vi "UDP Discover (subnet).vi"(0 "Name":string, 5 "receiver port":u16=10000, 7 "Excludes":string[](array[string]), 11 "error in (no error)":errorcluster) -> (4 "address:port":string, 6 "Address":string, 8 "Port":i32, 14 "local address":string, 15 "error out":errorcluster)   [LabVIEW 2020]
panel:
  in  "timeout ms (500)":i32=500
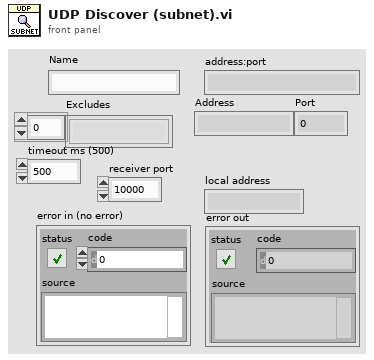
[diagram p1: front panel]
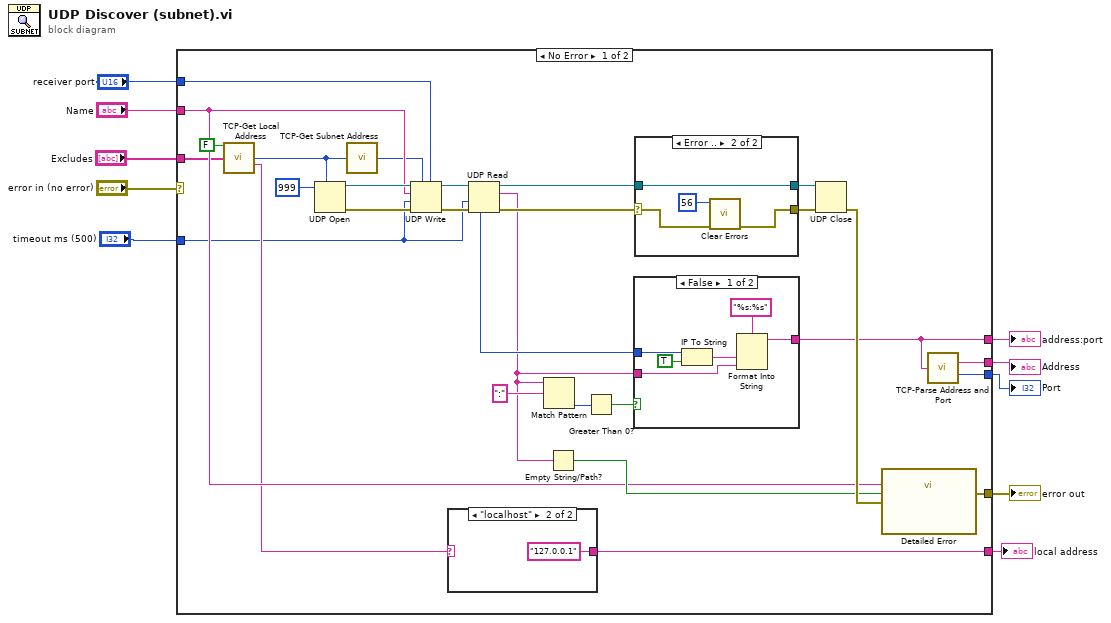
[diagram p0: block diagram]
diagram:
  n1 = case shown="No Error" "error in (no error)" {
    selector: "error in (no error)" -> [_ w55]
    tunnel: "receiver port" -> [w39 _]
    tunnel: [w24 _] -> w9
    tunnel: "Name" -> [w26 _]
    tunnel: [w25 w55] -> w7
    tunnel: [w23 _] -> w5
    tunnel: [w22 _] -> w4
    tunnel: [w20 _] -> w3
    tunnel: "Excludes" -> [w19 _]
    tunnel: "timeout ms (500)" -> [w11 _]
    frame No Error {
      n2 = call "TCP-Get Local Address.vi"("LAN first"=FALSE, "Excludes"=w19) -> ("net address"=w17:u32, "address"=w21:string)  [unwired: 12 in]
      n3 = UDP Open(7:w17, 11:u16 999 ("port")) -> (port=w37:refnum<k16>, 0:w38:errorcluster)  [unwired: 3 in, 1 out]
      n4 = call "TCP-Get Subnet Address.vi"("net address"=w17) -> ("subnet address"=w18:u32)  [unwired: 13 in, 1 out]
      n5 = UDP Write(address=w18, port or service name=w39, connection ID=w37, data in=w26, 8:w38, 9:w11) -> (error out=w34:errorcluster, 3:w31:refnum<k16>)
      n6 = case shown="\"localhost\"" w21 {
        selector: w21 -> [w40 _]
        tunnel: [w40 "127.0.0.1"] -> w20
        frame Default {
        }
        frame "localhost" {
        }
      }
      n7 = UDP Read(connection ID=w31, timeout ms (25000)=w11, 8:w34) -> (data out=w14:string, error out=w32:errorcluster, 3:w30:refnum<k16>, 6:w29:u32)  [unwired: 2 out]
      n8 = Match Pattern(string=w14, regular expression=":" ("search string/char (-)")) -> (offset past match=w13:i32)  [unwired: 1 in, 3 out]
      n9 = Empty String/Path?(string/path=w14) -> (empty?=w27:bool)
      n10 = Greater Than 0?(x=w13) -> (x > 0?=w12:bool)
      n11 = case shown="False" w12 {
        tunnel: w29 -> [w47 _]
        tunnel: [w43 w48] -> w24
        tunnel: w14 -> [w42 w48]
        frame False {
          n12 = IP To String(1:TRUE ("dot notation? (F)"), 2:w47) -> (0:w45:string)
          n13 = Format Into String(format string="%s:%s", w45, w42) -> (resulting string=w43:string)  [unwired: 2 in, 1 out]
        }
        frame True {
        }
      }
      n14 = case shown="Error .." w32 {
        selector: w32 -> [w49 w52]
        tunnel: w30 -> [w50 w54]
        tunnel: [w50 w54] -> w36
        tunnel: [w49 w51] -> w35
        frame No Error {
        }
        frame Error {
          n15 = call <vilib>:"Clear Errors.vi"("error in (no error)"=w52, "specific error code to clear (0: all)"=56) -> ("error out"=w51:errorcluster)  [unwired: 4 in, 1 out]
        }
      }
      n16 = UDP Close(connection ID=w36, 8:w35) -> (error out=w28:errorcluster)  [unwired: 1 out]
      n17 = call "Detailed Error"("Details"=w26, "Error?"=w27, "Primary"=w28) -> ("detailed error"=w25:errorcluster)  [unwired: 12 in]
      n18 = call "TCP-Parse Address and Port.vi"("Address in"=w24) -> ("Address"=w23:string, "Port"=w22:i32)  [unwired: 12 in, 1 out]
    }
    frame Error {
    }
  }
  "address:port" <- w9
  "error out" <- w7
  "Address" <- w5
  "Port" <- w4
  "local address" <- w3
